vi "CSU22 Parse Shutter Filter.vi"(0 "Reply String":string, 11 "Error In":errorcluster) -> (4 "Shutter Open?":bool, 8 "ND Filter Out?":bool, 15 "Error Out":errorcluster)   [LabVIEW 2020]
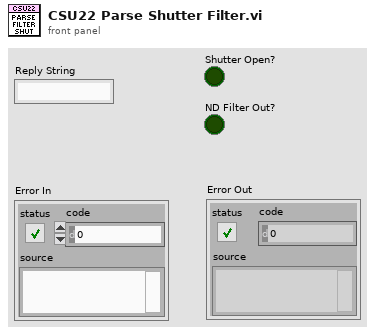
[diagram p1: front panel]
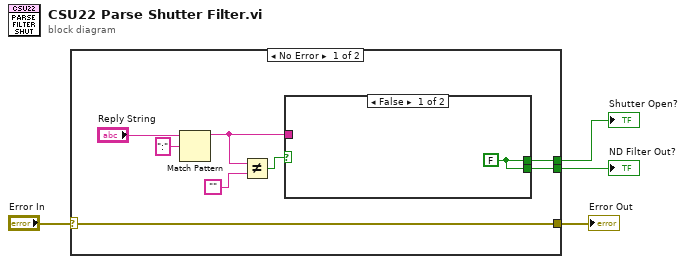
[diagram p0: block diagram]
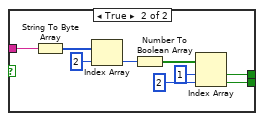
[diagram p2: hidden frame]
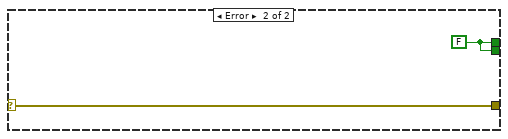
[diagram p3: hidden frame]
diagram:
  n1 = case shown="No Error" "Error In" {
    selector: "Error In" -> [w7 w24]
    tunnel: [w7 w24] -> w3
    tunnel: [w6 w23] -> w2
    tunnel: [w5 w23] -> w1
    frame No Error {
      n2 = Match Pattern(string="Reply String", regular expression=":") -> (before substring=w11:string)  [unwired: 1 in, 3 out]
      n3 = Not Equal?(x=w11, y="") -> (x != y?=w9:bool)
      n4 = case shown="False" w9 {
        tunnel: w11 -> [_ w19]
        tunnel: [w13 w15] -> w6
        tunnel: [w13 w14] -> w5
        frame False {
          w13 = FALSE
        }
        frame True {
          n5 = String To Byte Array(string=w19) -> (unsigned byte array=w22:u8[])
          n6 = Index Array(array=w22, index=2) -> (element=w20:u8)
          n7 = Number To Boolean Array(number=w20) -> (Boolean array=w18:bool[])
          n8 = Index Array(array=w18, index #1=1 ("index"), index #2=2 ("index")) -> (element #1=w15:bool, element #2=w14:bool)
        }
      }
    }
    frame Error {
      w23 = FALSE
    }
  }
  "Shutter Open?" <- w2
  "ND Filter Out?" <- w1
  "Error Out" <- w3
